vi "Coastdown.vi"(11 "Cluster":T1) -> (3 "Boolean":bool)   [LabVIEW 2013]
uses:
  Drive Train Metrics.ctl
  CmdFlag.ctl
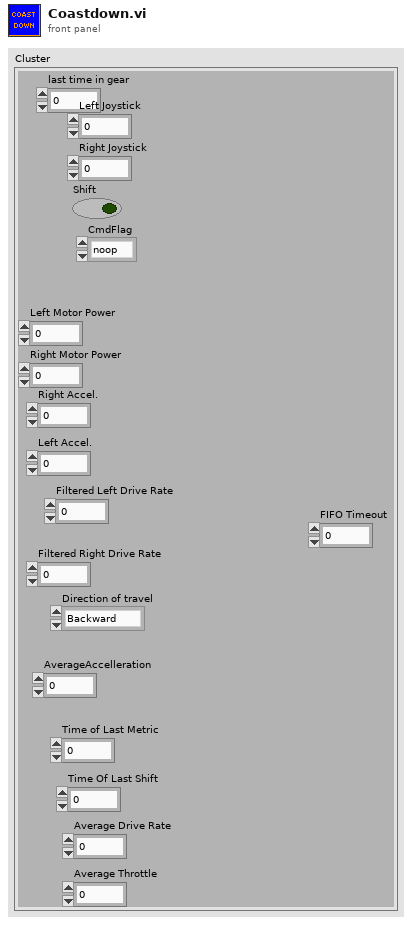
[diagram p1: front panel]
types:
  T1 = typedef "Drive Train Metrics.ctl" = cluster{"last time in gear":u32, "Shift":bool, "Right Joystick":dbl, "Left Joystick":dbl, "CmdFlag":T2, "Right Motor Power":dbl, "Left Motor Power":dbl, "Right Accel.":dbl, "Left Accel.":dbl, "Filtered Left Drive Rate":dbl, "Filtered Right Drive Rate":dbl, "Direction of travel":enum16{"Backward", "Forward", "Spin"}, "AverageAccelleration":dbl, "Time of Last Metric":u32, "Time Of Last Shift":dbl, "Average Drive Rate":dbl, "Average Throttle":dbl, "FIFO Timeout":i32}
  T2 = typedef "CmdFlag.ctl" = enum16{"noop", "suspend", "resume"}
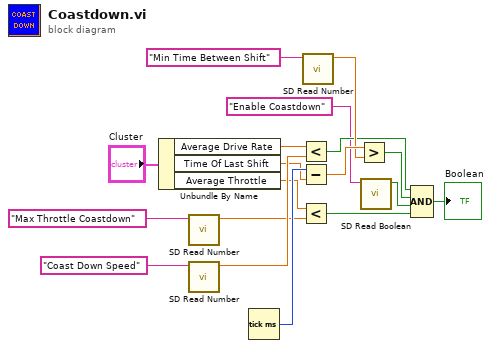
[diagram p0: block diagram]
diagram:
  n1 = Unbundle By Name("Cluster") -> ("Average Drive Rate"=w14:dbl, "Time Of Last Shift"=w12:dbl, "Average Throttle"=w2:dbl)
  n2 = call <vilib>:"SD Read Number.vi"("Name"="Max Throttle Coastdown") -> ("Numeric"=w3:dbl)  [unwired: 8 in, 2 out]
  n3 = call <vilib>:"SD Read Number.vi"("Name"="Coast Down Speed") -> ("Numeric"=w18:dbl)  [unwired: 8 in, 2 out]
  n4 = Tick Count (ms)() -> (millisecond timer value=w13:u32)
  n5 = Less?(x=w14, y=w18) -> (x < y?=w7:bool)
  n6 = Subtract(x=w13, y=w12) -> (x-y=w11:dbl)
  n7 = Less?(x=w2, y=w3) -> (x < y?=w1:bool)
  n8 = call <vilib>:"SD Read Number.vi"("Name"="Min Time Between Shift") -> ("Numeric"=w10:dbl)  [unwired: 8 in, 2 out]
  n9 = Greater?(x=w11, y=w10) -> (0:w8:bool)
  n10 = call <vilib>:"SD Read Boolean.vi"("Name"="Enable Coastdown") -> ("Boolean"=w6:bool)  [unwired: 8 in, 2 out]
  n11 = Compound Arithmetic op=AND(w7, w8, w6, w1) -> (→"Boolean":bool)
